vi "range_check_doubles.vi"(1 "high_limit":dbl, 2 "value":dbl, 3 "range":dbl=1e-15, 4 "low_limit":dbl) -> (6 "in range?":bool)   [LabVIEW 2021]
doc: "This VI compares one number (doubles) and checks if it is inside a defined high and low limit.\nThe default range is set to 1 femto = 1E-15."
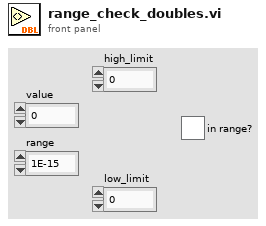
[diagram p1: front panel]
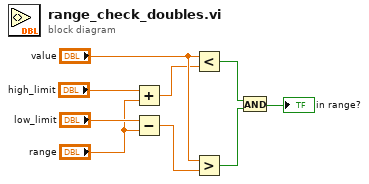
[diagram p0: block diagram]
diagram:
  n1 = Add(x="high_limit", y="range") -> (x+y=w5:dbl)
  n2 = Subtract(x="low_limit", y="range") -> (x-y=w4:dbl)
  n3 = Less?(x="value", y=w5) -> (x < y?=w3:bool)
  n4 = Greater?(x="value", y=w4) -> (0:w2:bool)
  n5 = And(x=w3, y=w2) -> (x .and. y?=→"in range?":bool)
